vi "Set calibration mode.vi"(8 "error in":errorcluster, 10 "Calibration mode (disable)":u16(ring) items=["Disable", "Enable"], 11 "VISA resource name":refnum<visa-resource-name>) -> (0 "error out":errorcluster, 3 "VISA resource name out":refnum<visa-resource-name>)   [LabVIEW 2012, in "Datron D4xxx.lvlib"]
doc: "This VI enables/disables calibration mode. It can be enabeld only if key is in \"calibration enable\" position."
uses:
  Datron D4xxx.lvlib
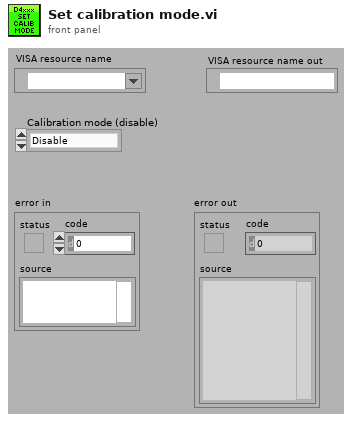
[diagram p1: front panel]
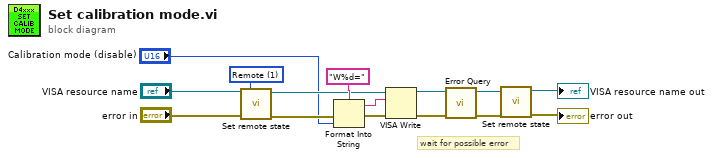
[diagram p0: block diagram]
diagram:
  w2 = u16 1 items=["Local", "Remote", "Default"] ("Remote state")
  # "wait for possible error"
  n1 = call "Set remote state.vi"("error in"="error in", "Remote state"=w2, "VISA resource name"="VISA resource name") -> ("error out"=w5:errorcluster, "VISA resource name out"=w3:refnum<visa-resource-name>)  [unwired: 7 in]
  n2 = Format Into String(format string="W%d=", error in=w5, "Calibration mode (disable)") -> (resulting string=w15:string, error out=w14:errorcluster)  [unwired: 1 in]
  n3 = VISA Write(VISA resource name=w3, write buffer=w15, error in (no error)=w14) -> (VISA resource name out=w7:refnum<visa-resource-name>, error out=w8:errorcluster)  [unwired: 1 out]
  n4 = call "Error Query.vi"("error in (no error)"=w8, "VISA resource name"=w7) -> ("error out"=w12:errorcluster, "VISA resource name out"=w10:refnum<visa-resource-name>)  [unwired: 6 in, 2 out]
  n5 = call "Set remote state.vi"("error in"=w12, "VISA resource name"=w10) -> ("error out"=→"error out":errorcluster, "VISA resource name out"=→"VISA resource name out":refnum<visa-resource-name>)  [unwired: 8 in]
